vi "Simulation Record Get.vi"(8 "Error In":errorcluster, 11 "simulator":T17={"configuration"={"maxTime"=5.0, "enableVisualization"=TRUE, "statechart"=path "iRobot Navigation State Machine.vi", "environment"=path "iRobot Navigation State Machine.vi", "record"=path "Simulation Record.xml", "autograde?"=TRUE, "interactive?"=FALSE, "feedback mode"=enum."debug navigation"}, "Bump Sensors"=[], "Distance Sensors"=[], "Accelerometer"=refnum, "Wall Sensor"=refnum, "Statechart\ndisplay"=refnum, "Body"=refnum, "Left Motor"=refnum, "Right Motor"=refnum, "first step?"=FALSE}) -> (0 "Error Out":errorcluster, 2 "record":T1={"configuration"={"maxTime"=5.0, "enableVisualization"=TRUE, "statechart"=path "iRobot Navigation State Machine.vi", "environment"=path "iRobot Navigation State Machine.vi", "record"=path "Simulation Record.xml", "autograde?"=TRUE, "interactive?"=FALSE, "feedback mode"=enum."debug navigation"}, "trace"=[], "environment MD5"="", "statechart MD5"="", "record timestamp"=""} {"trace"."sensors"."iRobot Sensors"."Infrared" format="%02x"; "trace"."sensors"."accelerometer"."z axis (g)" format="%.3f"; "trace"."sensors"."accelerometer"."y axis (g)" format="%.3f"; "trace"."sensors"."accelerometer"."x axis (g)" format="%.3f"}, 3 "simulator":T17={"configuration"={"maxTime"=5.0, "enableVisualization"=TRUE, "statechart"=path "iRobot Navigation State Machine.vi", "environment"=path "iRobot Navigation State Machine.vi", "record"=path "Simulation Record.xml", "autograde?"=TRUE, "interactive?"=FALSE, "feedback mode"=enum."debug navigation"}, "Bump Sensors"=[], "Distance Sensors"=[], "Accelerometer"=refnum, "Wall Sensor"=refnum, "Statechart\ndisplay"=refnum, "Body"=refnum, "Left Motor"=refnum, "Right Motor"=refnum, "first step?"=FALSE})   [LabVIEW 2013]
uses:
  Simulator.ctl
  <instrlib>/DC Motor Controller/HAIOL/DC Motor Controller.lvclass
  CyberSim interface/Simulation Configuration.ctl
  autograder/feedbackMode.ctl
  Simulation Record.ctl
  Simulation Trace Element.ctl
  shared/Sensors.ctl
  iRobot/Sensor/Accelerometer.ctl
  iRobot/Sensor/Sensor Group 6.ctl
  iRobot/Sensor/Bumps + Wheel Drops.ctl
  iRobot/Sensor/Buttons.ctl
  iRobot/Sensor/Charging State.ctl
  iRobot/Sensor/Charging Sources Available.ctl
  iRobot/Sensor/OI Mode.ctl
  iRobot/Sensor/Cargo Bay Digital Inputs.ctl
  iRobot/Sensor/Low-Side Driver + Wheel Overcurrent.ctl
  Simulated iRobot Position.ctl
  Simulated iRobot Orientation.ctl
  Simulation Trace Operation.ctl
panel:
  # "Electrical: charging, battery, OI mode"
  # "Sensors: bump, cliff, button, wheel drop, wall, virtual wall"
  # "Motion: distance, angle, requested velocity"
  # "Cargo Bay: I/O, overcurrent, infrared"
  # "Song"
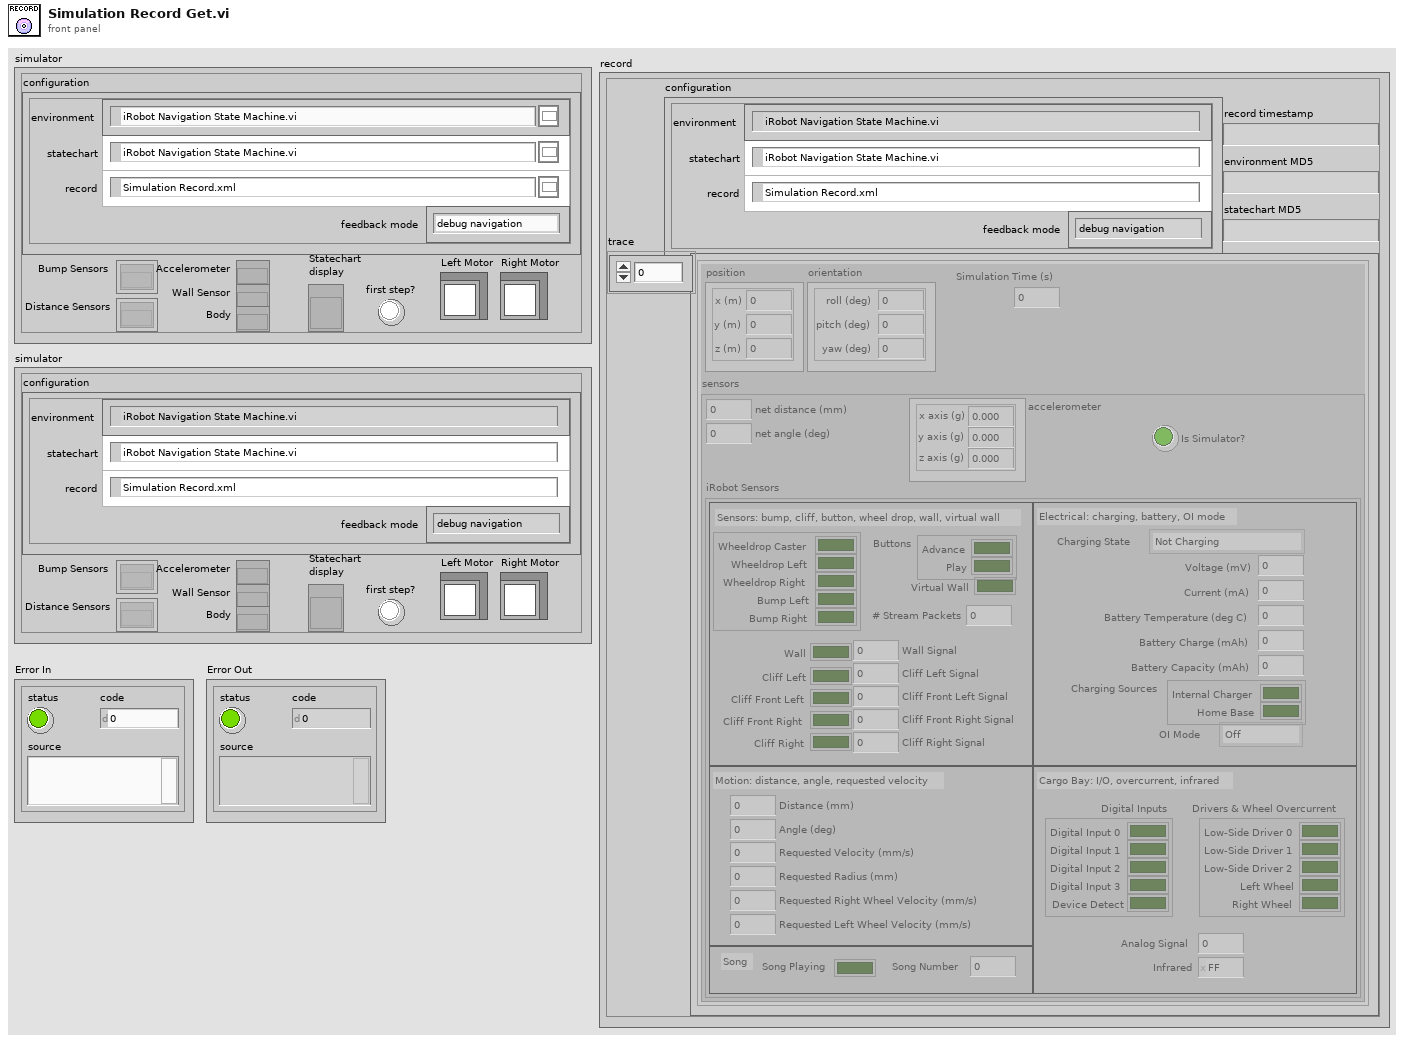
[diagram p1: front panel]
types:
  T1 = typedef "Simulation Record.ctl" = cluster{"configuration":T2, "trace":T4[], "environment MD5":string, "statechart MD5":string, "record timestamp":string}
  T2 = typedef "Simulation Configuration.ctl" = cluster{"maxTime":sgl, "enableVisualization":bool, "statechart":path, "environment":path, "record":path, "autograde?":bool, "interactive?":bool, "feedback mode":T3}
  T3 = typedef "feedbackMode.ctl" = enum32{"debug navigation", "debug hill climb", "autograde navigation", "autograde hill climb"}
  T4 = typedef "Simulation Trace Element.ctl" = cluster{"sensors":T5, "position":T15, "orientation":T16, "Simulation Time (s)":sgl}
  T5 = typedef "Sensors.ctl" = cluster{"net distance (mm)":i32, "net angle (deg)":i32, "accelerometer":T6, "iRobot Sensors":T7, "Is Simulator?":bool}
  T6 = typedef "Accelerometer.ctl" = cluster{"x axis (g)":dbl, "y axis (g)":dbl, "z axis (g)":dbl}
  T7 = typedef "Sensor Group 6.ctl" = cluster{"Bumps + Wheel Drops":T8, "Wall":bool, "Cliff Left":bool, "Cliff Front Left":bool, "Cliff Front Right":bool, "Cliff Right":bool, "Wall Signal":u16, "Cliff Left Signal":u16, "Cliff Front Left Signal":u16, "Cliff Front Right Signal":u16, "Cliff Right Signal":u16, "Buttons":T9, "Virtual Wall":bool, "# Stream Packets":u8, "Requested Velocity (mm/s)":i16, "Requested Radius (mm)":i16, "Requested Right Wheel Velocity (mm/s)":i16, "Requested Left Wheel Velocity (mm/s)":i16, "Distance (mm)":i32, "Angle (deg)":i32, "Song Playing":bool, "Song Number":u8, "Charging State":T10, "Voltage (mV)":u16, "Current (mA)":i16, "Battery Temperature (deg C)":i8, "Battery Charge (mAh)":u16, "Battery Capacity (mAh)":u16, "Charging Sources":T11, "OI Mode":T12, "Digital Inputs":T13, "Drivers & Wheel Overcurrent":T14, "Analog Signal":u16, "Infrared":u8}
  T8 = typedef "Bumps + Wheel Drops.ctl" = cluster{"Wheeldrop Caster":bool, "Wheeldrop Left":bool, "Wheeldrop Right":bool, "Bump Left":bool, "Bump Right":bool}
  T9 = typedef "Buttons.ctl" = cluster{"Advance":bool, "Play":bool}
  T10 = typedef "Charging State.ctl" = enum16{"Not Charging", "Reconditioning Charging", "Full Charging", "Trickle Charging", "Waiting", "Charging Fault Condition"}
  T11 = typedef "Charging Sources Available.ctl" = cluster{"Internal Charger":bool, "Home Base":bool}
  T12 = typedef "OI Mode.ctl" = enum16{"Off", "Passive", "Safe", "Full"}
  T13 = typedef "Cargo Bay Digital Inputs.ctl" = cluster{"Digital Input 0":bool, "Digital Input 1":bool, "Digital Input 2":bool, "Digital Input 3":bool, "Device Detect":bool}
  T14 = typedef "Low-Side Driver + Wheel Overcurrent.ctl" = cluster{"Low-Side Driver 0":bool, "Low-Side Driver 1":bool, "Low-Side Driver 2":bool, "Left Wheel":bool, "Right Wheel":bool}
  T15 = typedef "Simulated iRobot Position.ctl" = cluster{"x (m)":sgl, "y (m)":sgl, "z (m)":sgl}
  T16 = typedef "Simulated iRobot Orientation.ctl" = cluster{"roll (deg)":sgl, "pitch (deg)":sgl, "yaw (deg)":sgl}
  T17 = typedef "Simulator.ctl" = cluster{"configuration":T2, "Bump Sensors":refnum<k20>[], "Distance Sensors":refnum<k20>[], "Accelerometer":refnum<k20>, "Wall Sensor":refnum<k20>, "Statechart\ndisplay":refnum<vi>, "Body":refnum<k20>, "Left Motor":refnum<class "DC Motor Controller.lvclass">, "Right Motor":refnum<class "DC Motor Controller.lvclass">, "first step?":bool}
  T18 = typedef "Simulation Trace Operation.ctl" = enum16{"Initialize", "Record Trace Element", "Get Trace"}
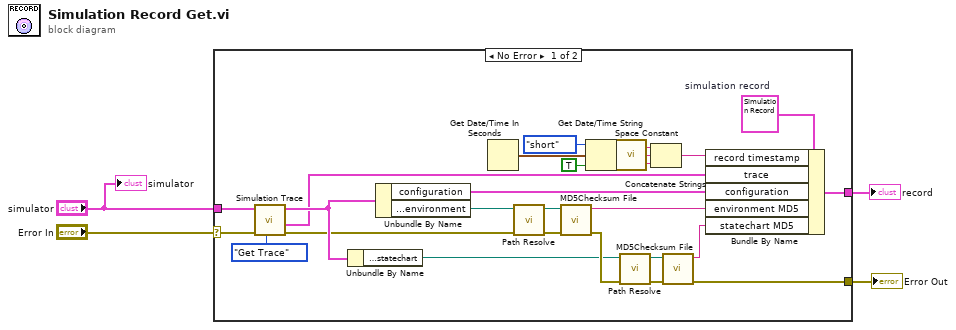
[diagram p0: block diagram]
diagram:
  n1 = case shown="No Error" "Error In" {
    selector: "Error In" -> [w5 w31]
    tunnel: [w30 w31] -> w4
    tunnel: "simulator" -> [w29 _]
    tunnel: [w28 _] -> w3
    frame No Error {
      w26 = T1 {"configuration"={"maxTime"=0.0, "enableVisualization"=FALSE, "statechart"=path "", "environment"=path "", "record"=path "", "autograde?"=FALSE, "interactive?"=FALSE, "feedback mode"=enum."debug navigation"}, "trace"=[], "environment MD5"="", "statechart MD5"="", "record timestamp"=""}  # simulation record
      n2 = call "Simulation Trace.vi"("operation"=Simulation_Trace_Operation."Get Trace", "error in"=w5, "simulator"=w29) -> ("error out"=w17:errorcluster, "trace"=w21:T4[], "simulator"=w27:T17)  [unwired: 5 in, 1 out]
      n3 = Unbundle By Name(w27) -> ("configuration.statechart"=w13:path)
      n4 = Unbundle By Name(w27) -> ("configuration"=w23:T2, "configuration.environment"=w18:path)
      n5 = Get Date/Time In Seconds() -> (seconds since 1Jan1904=w7:timestamp)
      n6 = call "Path Resolve.vi"("Error In"=w17, "absolute or relative path"=w18) -> ("Error Out"=w20:errorcluster, "resolved path"=w19:path)  [unwired: 8 in]
      n7 = call <vilib>:"MD5Checksum File.vi"("error in (no error)"=w20, "Path"=w19) -> ("error out"=w14:errorcluster, "MD5 message-digest"=w25:string)  [unwired: 8 in]
      n8 = Get Date/Time String(date format (0)=enum16{"short", "long", "abbreviated"}."short", seconds (now)=w7, want seconds? (F)=TRUE) -> (date string=w10:string, time string=w9:string)
      n9 = call <vilib>:"Space Constant.vi"() -> ("String"=w8:string)
      n10 = call "Path Resolve.vi"("Error In"=w14, "absolute or relative path"=w13) -> ("Error Out"=w15:errorcluster, "resolved path"=w16:path)  [unwired: 8 in]
      n11 = Concatenate Strings(w10, w8, w9) -> (w6:string)
      n12 = call <vilib>:"MD5Checksum File.vi"("error in (no error)"=w15, "Path"=w16) -> ("error out"=w30:errorcluster, "MD5 message-digest"=w24:string)  [unwired: 8 in]
      n13 = Bundle By Name(cluster=w26, "record timestamp"=w6, "trace"=w21, "configuration"=w23, "environment MD5"=w25, "statechart MD5"=w24) -> (w28:T1)
    }
    frame Error {
    }
  }
  "Error Out" <- w4
  "record" <- w3
  "simulator" <- "simulator"
